vi "MessageName.vi"() -> (2 "MessageName":string)   [LabVIEW 2020, in "StopLog.lvlib"]
uses:
  StopLog.lvlib
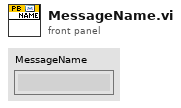
[diagram p1: front panel]
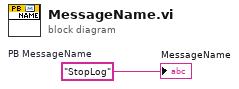
[diagram p0: block diagram]
diagram:
  w1 = "StopLog"  # PB MessageName
  "MessageName" <- w1
